vi "SP Calculate SXX.vi"(10 "TP Array (TXX, TXY, TYX, TYY)":cdb[](array[numeric])) -> (2 "SXX":cdb)   [LabVIEW 2011]
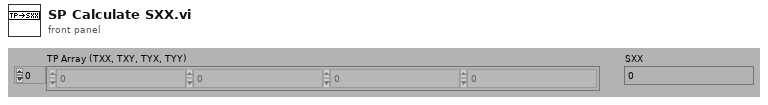
[diagram p1: front panel]
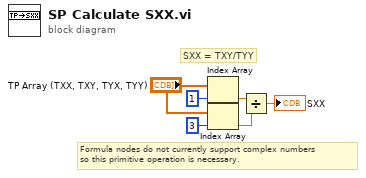
[diagram p0: block diagram]
diagram:
  # "SXX = TXY/TYY"
  # "Formula nodes do not currently support complex numbers\nso this primitive operation is necessary."
  n1 = Index Array(array="TP Array (TXX, TXY, TYX, TYY)", index=1) -> (element=w3:cdb)
  n2 = Index Array(array="TP Array (TXX, TXY, TYX, TYY)", index=3) -> (element=w2:cdb)
  n3 = Divide(x=w3, y=w2) -> (x/y=→"SXX":cdb)
